vi "GetParam.vi"(8 "error in (no error)":errorcluster caption="entrée d'erreur (pas d'erreur)", 11 "Zero_One_Loss.lvclass":refnum<class "Zero_One_Loss.lvclass">) -> (0 "error out":errorcluster caption="sortie d'erreur", 2 "zero_one_loss":cluster{"normalize":bool, "sample_weight":dbl[]}={"normalize"=TRUE, "sample_weight"=[]}, 3 "Zero_One_Loss.lvclass":refnum<class "Zero_One_Loss.lvclass">)   [LabVIEW 2020, in "Zero_One_Loss.lvclass"]
doc: "Get Parameters"
uses:
  Zero_One_Loss.lvclass
  Zero_One_Loss.lvclass/Zero_One_Loss.ctl
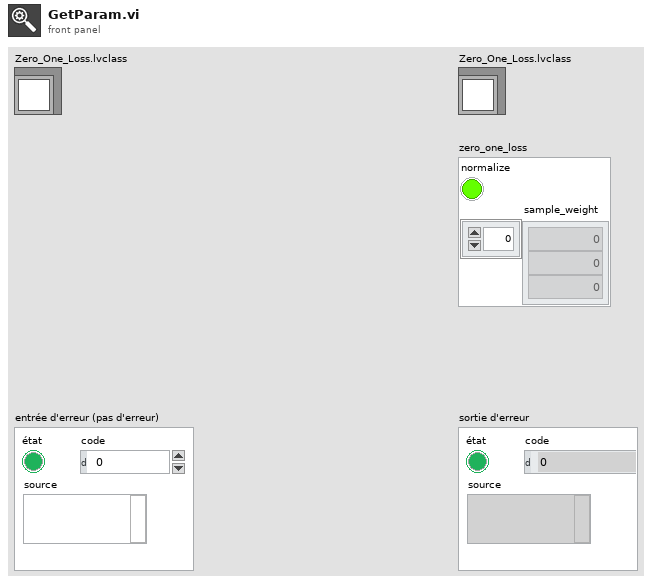
[diagram p1: front panel]
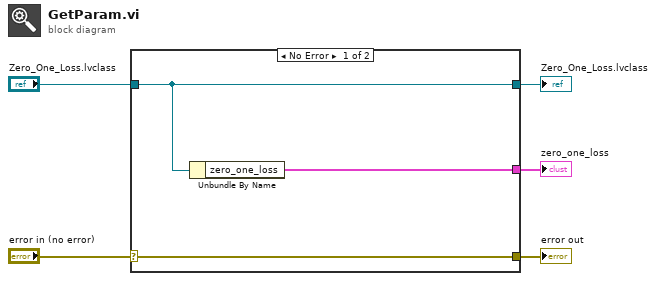
[diagram p0: block diagram]
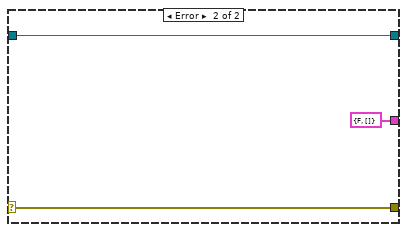
[diagram p2: hidden frame]
diagram:
  n1 = case shown="No Error" "error in (no error)" {
    selector: "error in (no error)" -> [w8 w10]
    tunnel: [w8 w10] -> w4
    tunnel: [w7 w11] -> w2
    tunnel: "Zero_One_Loss.lvclass" -> [w7 w11]
    tunnel: [w6 cluster{"normalize":bool, "sample_weight":dbl[]} {"normalize"=FALSE, "sample_weight"=[]} ("zero_one_loss")] -> w1
    frame No Error {
      n2 = Unbundle By Name(w7) -> ("zero_one_loss"=w6:cluster{"normalize":bool, "sample_weight":dbl[]})
    }
    frame Error {
    }
  }
  "error out" <- w4
  "Zero_One_Loss.lvclass" <- w2
  "zero_one_loss" <- w1
